vi "Get UI Refs.vi"(8 "error in (no error)":errorcluster, 11 "VI Refnum":refnum<vi>) -> (0 "error out":errorcluster, 3 "UI References":T1)   [LabVIEW 2018, in "Numeric Data Type.lvclass"]
uses:
  Numeric Data Type.lvclass
  UI References.ctl
  Representation Ring.ctl
  <vilib>/fxp/FXPxcontrol/FXP.xctl
  Response to Values Outside of Limits Enum.ctl
  Precision Type.ctl
  Padding.ctl
  Time Format.ctl
  Clock Type.ctl
  Date Format.ctl
  Date Order.ctl
  Year Format.ctl
  Format Code Type List Enum.ctl
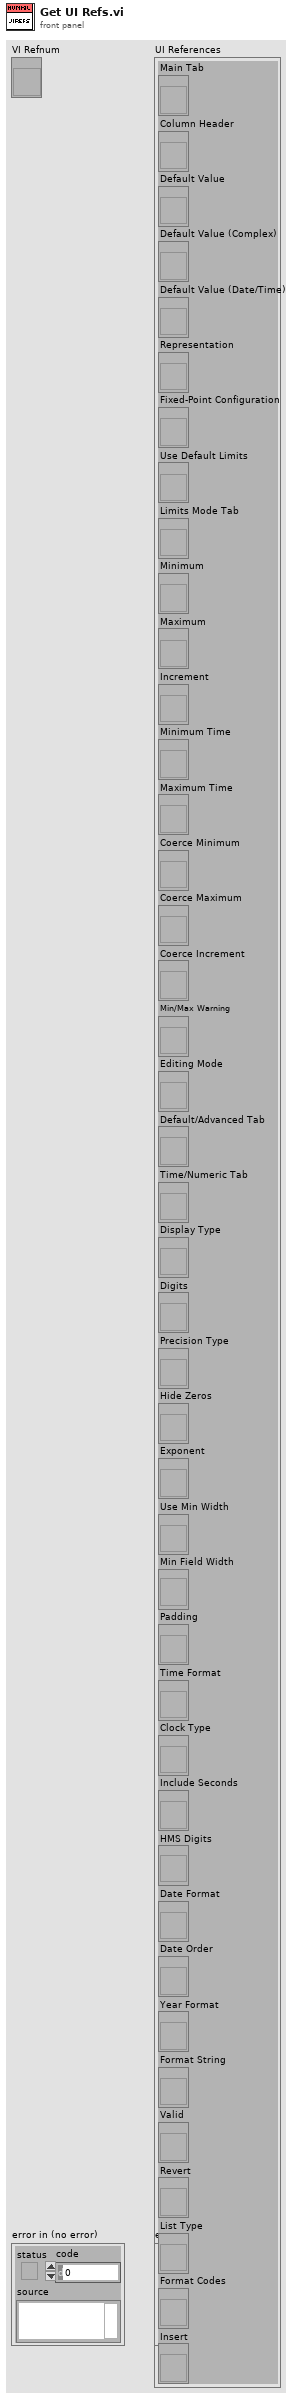
[diagram p1: front panel]
types:
  T1 = typedef "Numeric Data Type.lvclass/UI References.ctl" = cluster{"Main Tab":refnum<vi>, "Column Header":refnum<vi>, "Default Value":refnum<vi>, "Default Value (Complex)":refnum<vi>, "Default Value (Date/Time)":refnum<vi>, "Representation":refnum<vi>, "Fixed-Point Configuration":refnum<vi>, "Use Default Limits":refnum<vi>, "Limits Mode Tab":refnum<vi>, "Minimum":refnum<vi>, "Maximum":refnum<vi>, "Increment":refnum<vi>, "Minimum Time":refnum<vi>, "Maximum Time":refnum<vi>, "Coerce Minimum":refnum<vi>, "Coerce Maximum":refnum<vi>, "Coerce Increment":refnum<vi>, "Min/Max Warning":refnum<vi>, "Editing Mode":refnum<vi>, "Default/Advanced Tab":refnum<vi>, "Time/Numeric Tab":refnum<vi>, "Display Type":refnum<vi>, "Digits":refnum<vi>, "Precision Type":refnum<vi>, "Hide Zeros":refnum<vi>, "Exponent":refnum<vi>, "Use Min Width":refnum<vi>, "Min Field Width":refnum<vi>, "Padding":refnum<vi>, "Time Format":refnum<vi>, "Clock Type":refnum<vi>, "Include Seconds":refnum<vi>, "HMS Digits":refnum<vi>, "Date Format":refnum<vi>, "Date Order":refnum<vi>, "Year Format":refnum<vi>, "Format String":refnum<vi>, "Valid":refnum<vi>, "Revert":refnum<vi>, "List Type":refnum<vi>, "Format Codes":refnum<vi>, "Insert":refnum<vi>}
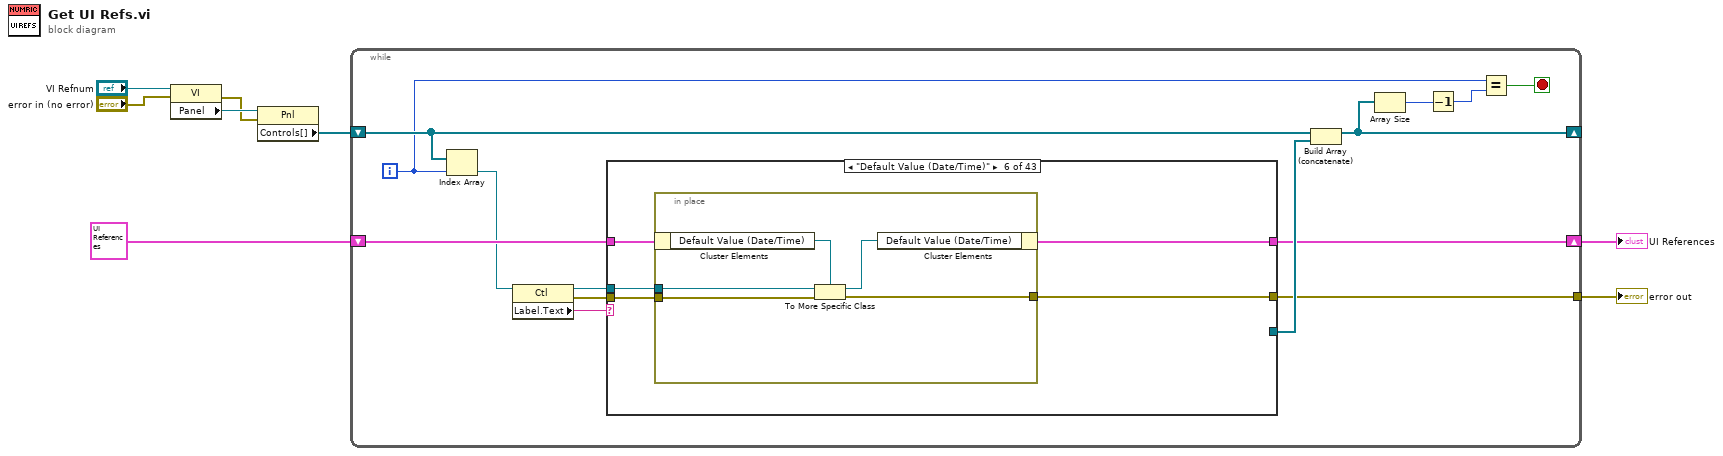
[diagram p0: block diagram]
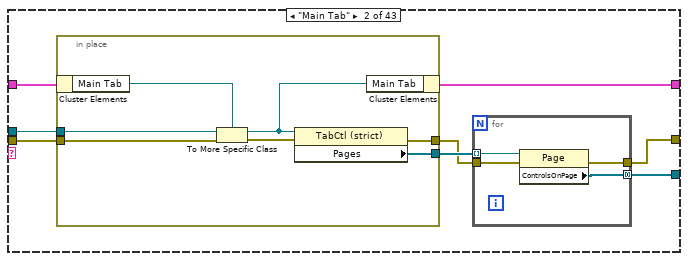
[diagram p3: hidden frame]
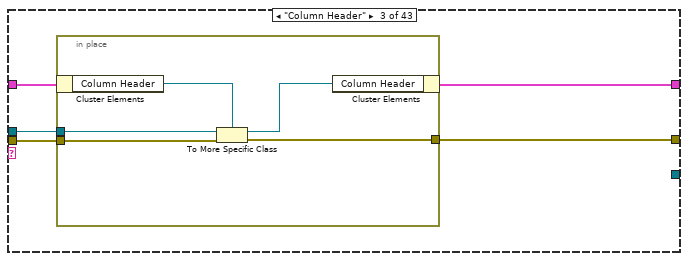
[diagram p4: hidden frame]
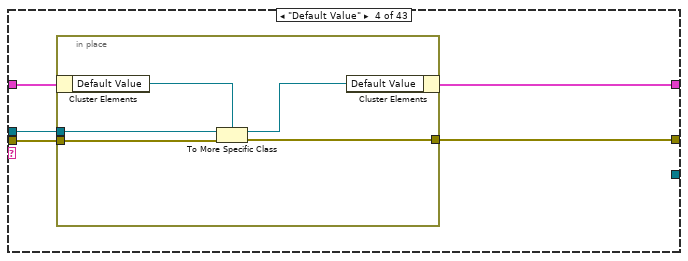
[diagram p5: hidden frame]
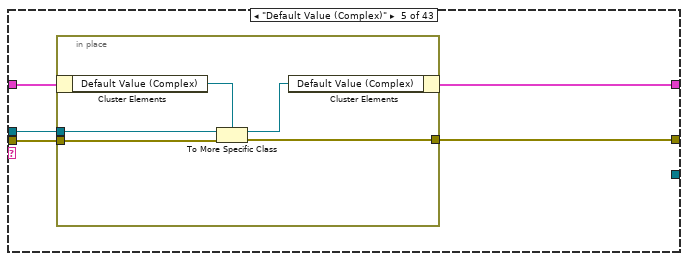
[diagram p6: hidden frame]
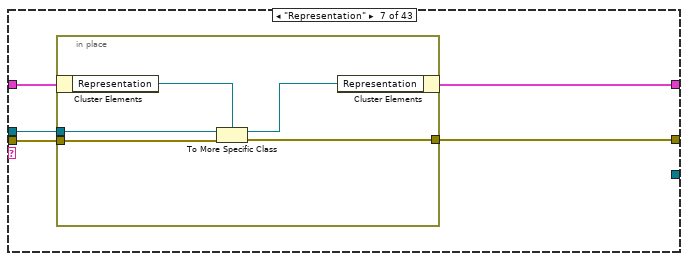
[diagram p7: hidden frame]
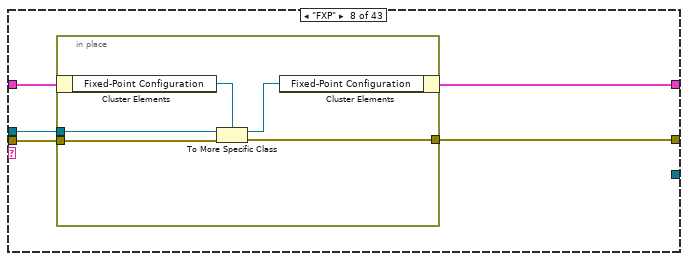
[diagram p8: hidden frame]
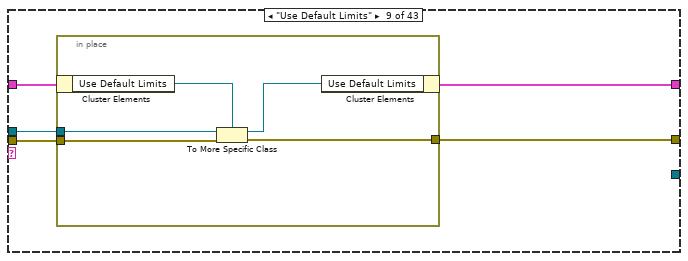
[diagram p9: hidden frame]
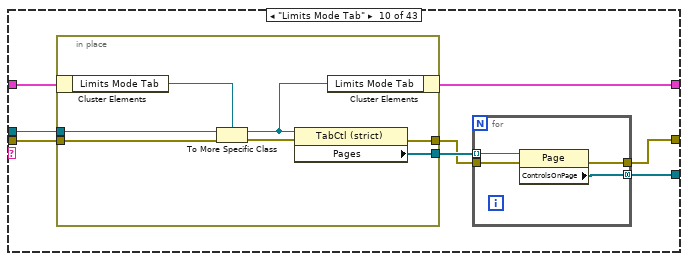
[diagram p10: hidden frame]
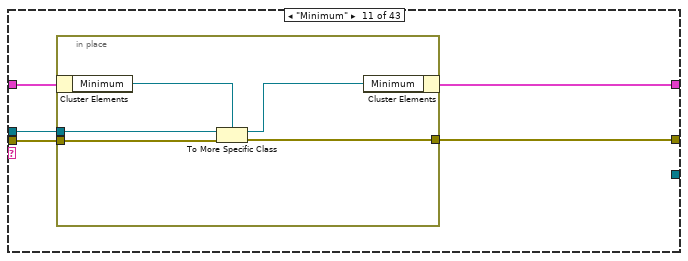
[diagram p11: hidden frame]
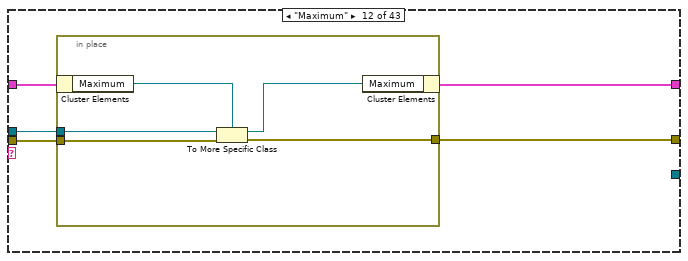
[diagram p12: hidden frame]
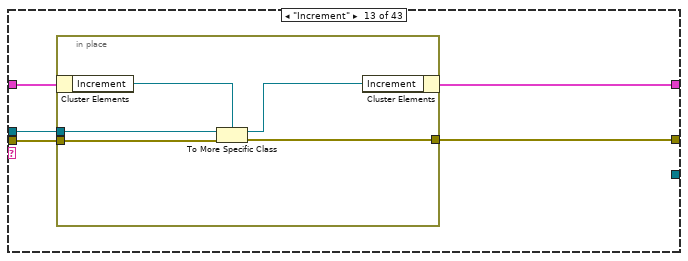
[diagram p13: hidden frame]
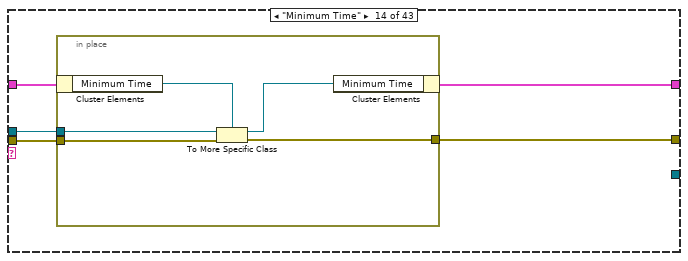
[diagram p14: hidden frame]
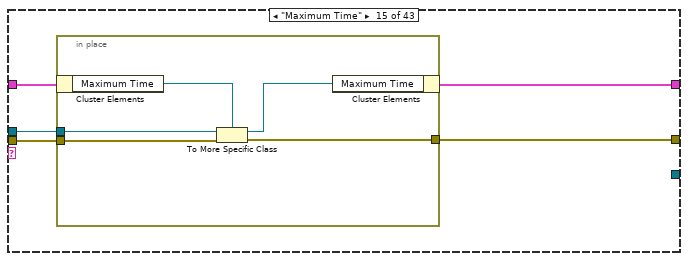
[diagram p15: hidden frame]
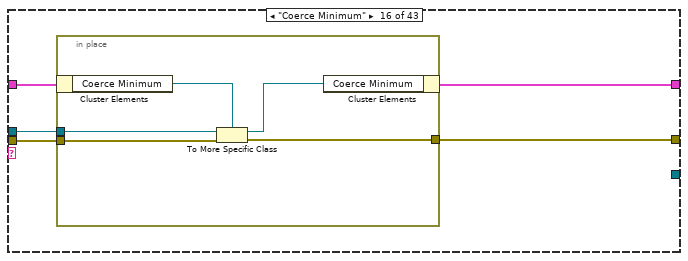
[diagram p16: hidden frame]
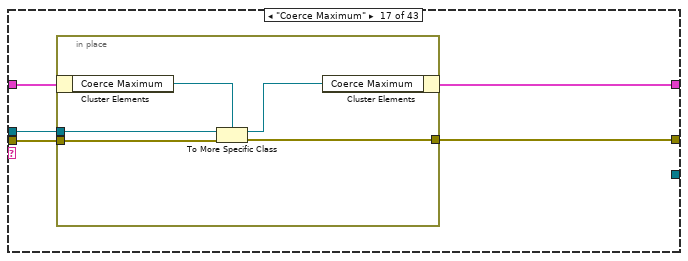
[diagram p17: hidden frame]
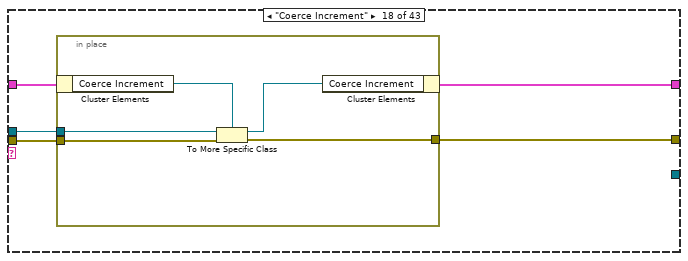
[diagram p18: hidden frame]
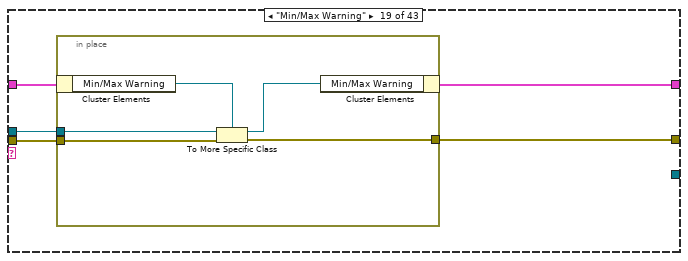
[diagram p19: hidden frame]
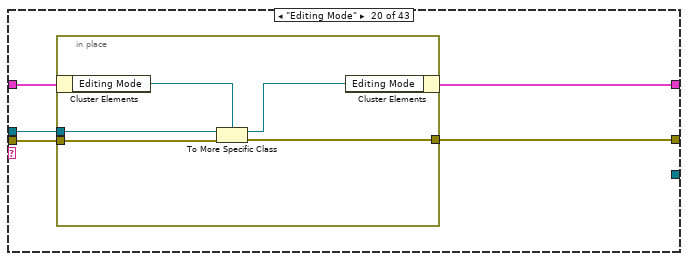
[diagram p20: hidden frame]
diagram:
  n1 = property class="VI"(reference="VI Refnum", error in="error in (no error)") -> (error out=w1:errorcluster, "Panel"=w4:refnum<vi>)  [unwired: 1 out]
  n2 = property class="Pnl"(reference=w4, error in=w1) -> ("Controls[]"=w3:refnum<vi>[])  [unwired: 2 out]
  n3 = while {
    shift-right: [w10] -> w6
    shift-left: T1 {"Main Tab"=refnum, "Column Header"=refnum, "Default Value"=refnum, "Default Value (Complex)"=refnum, "Default Value (Date/Time)"=refnum, "Representation"=refnum, "Fixed-Point Configuration"=refnum, "Use Default Limits"=refnum, "Limits Mode Tab"=refnum, "Minimum"=refnum, "Maximum"=refnum, "Increment"=refnum, "Minimum Time"=refnum, "Maximum Time"=refnum, "Coerce Minimum"=refnum, "Coerce Maximum"=refnum, "Coerce Increment"=refnum, "Min/Max Warning"=refnum, "Editing Mode"=refnum, "Default/Advanced Tab"=refnum, "Time/Numeric Tab"=refnum, "Display Type"=refnum, "Digits"=refnum, "Precision Type"=refnum, "Hide Zeros"=refnum, "Exponent"=refnum, "Use Min Width"=refnum, "Min Field Width"=refnum, "Padding"=refnum, "Time Format"=refnum, "Clock Type"=refnum, "Include Seconds"=refnum, "HMS Digits"=refnum, "Date Format"=refnum, "Date Order"=refnum, "Year Format"=refnum, "Format String"=refnum, "Valid"=refnum, "Revert"=refnum, "List Type"=refnum, "Format Codes"=refnum, "Insert"=refnum} ("UI References") -> [w22]
    shift-right: [w15] -> _
    shift-left: w3 -> [w17]
    tunnel: [w9] -> w8
    i -> [w13]
    stop <- w11 stop-if-true
    n4 = Index Array(array=w17, index=w13) -> (element=w21:refnum<vi>)
    n5 = property class="Ctl"(reference=w21) -> (reference out=w19:refnum<vi>, error out=w18:errorcluster, "Label.Text"=w20:string)  [unwired: 1 in]
    n6 = case shown="\"Default Value (Date/Time)\"" w20 {
      tunnel: w22 -> [w24 w31 w47 w57 w67 w77 w87 w97 w107 w120 w136 w146 w156 w166 w176 w186 w196 w206 w216 w226 w239 w258 w274 w284 w294 w304 w314 w324 w334 w344 w354 w364 w374 w384 w394 w404 w414 w424 w434 w444 w454 w464 w474]
      tunnel: w19 -> [_ w32 w48 w58 w68 w78 w88 w98 w108 w121 w137 w147 w157 w167 w177 w187 w197 w207 w217 w227 w240 w259 w275 w285 w295 w305 w315 w325 w335 w345 w355 w365 w375 w385 w395 w405 w415 w425 w435 w445 w455 w465 w475]
      tunnel: w18 -> [w23 w30 w46 w56 w66 w76 w86 w96 w106 w119 w135 w145 w155 w165 w175 w185 w195 w205 w215 w225 w238 w257 w273 w283 w293 w303 w313 w323 w333 w343 w353 w363 w373 w383 w393 w403 w413 w423 w433 w443 w453 w463 w473]
      tunnel: [_ w28 _ _ _ _ _ _ _ w117 _ _ _ _ _ _ _ _ _ _ w236 w255 _ _ _ _ _ _ _ _ _ _ _ _ _ _ _ _ _ _ _ _ _] -> w16
      tunnel: [w24 w27 w45 w55 w65 w75 w85 w95 w105 w116 w134 w144 w154 w164 w174 w184 w194 w204 w214 w224 w235 w254 w272 w282 w292 w302 w312 w322 w332 w342 w352 w362 w372 w382 w392 w402 w412 w422 w432 w442 w452 w462 w472] -> w10
      tunnel: [w23 w25 w44 w54 w64 w74 w84 w94 w104 w114 w133 w143 w153 w163 w173 w183 w193 w203 w213 w223 w233 w252 w271 w281 w291 w301 w311 w321 w331 w341 w351 w361 w371 w381 w391 w401 w411 w421 w431 w441 w451 w461 w471] -> w9
      frame Default {
      }
      frame "Main Tab" {
        n7 = in-place {
          in-place-border: w32 -> [w39]
          in-place-border: w30 -> [w37]
          in-place-border: [w34] -> w29
          in-place-border: [w33] -> w26
          n8 = in-place-cluster #1(w31) -> ("Main Tab"=w38:refnum<vi>)
          n9 = To More Specific Class(target class=w38, reference=w39, error in=w37) -> (specific class reference=w36:refnum<vi>, error out=w35:errorcluster)
          n10 = property class="TabCtl (strict)"(reference=w36, error in=w35) -> (error out=w33:errorcluster, "Pages"=w34:refnum<vi>[])  [unwired: 1 out]
          n11 = in-place-cluster #1("Main Tab"=w36) -> (w27:T1)
        }
        n12 = for {
          tunnel: w29 -> [w43] mode=indexing
          tunnel: [w42] -> w28 mode=concatenating
          tunnel: w26 -> [w41]
          tunnel: [w40] -> w25
          n13 = property class="Page"(reference=w43, error in=w41) -> (error out=w40:errorcluster, "ControlsOnPage"=w42:refnum<vi>[])  [unwired: 1 out]
        }
      }
      frame "Column Header" {
        n14 = in-place {
          in-place-border: w48 -> [w53]
          in-place-border: w46 -> [w51]
          in-place-border: [w49] -> w44
          n15 = in-place-cluster #2(w47) -> ("Column Header"=w52:refnum<vi>)
          n16 = To More Specific Class(target class=w52, reference=w53, error in=w51) -> (specific class reference=w50:refnum<vi>, error out=w49:errorcluster)
          n17 = in-place-cluster #2("Column Header"=w50) -> (w45:T1)
        }
      }
      frame "Default Value" {
        n18 = in-place {
          in-place-border: w58 -> [w63]
          in-place-border: w56 -> [w61]
          in-place-border: [w59] -> w54
          n19 = in-place-cluster #3(w57) -> ("Default Value"=w62:refnum<vi>)
          n20 = To More Specific Class(target class=w62, reference=w63, error in=w61) -> (specific class reference=w60:refnum<vi>, error out=w59:errorcluster)
          n21 = in-place-cluster #3("Default Value"=w60) -> (w55:T1)
        }
      }
      frame "Default Value (Complex)" {
        n22 = in-place {
          in-place-border: w68 -> [w73]
          in-place-border: w66 -> [w71]
          in-place-border: [w69] -> w64
          n23 = in-place-cluster #4(w67) -> ("Default Value (Complex)"=w72:refnum<vi>)
          n24 = To More Specific Class(target class=w72, reference=w73, error in=w71) -> (specific class reference=w70:refnum<vi>, error out=w69:errorcluster)
          n25 = in-place-cluster #4("Default Value (Complex)"=w70) -> (w65:T1)
        }
      }
      frame "Default Value (Date/Time)" {
        n26 = in-place {
          in-place-border: w78 -> [w83]
          in-place-border: w76 -> [w81]
          in-place-border: [w79] -> w74
          n27 = in-place-cluster #5(w77) -> ("Default Value (Date/Time)"=w82:refnum<vi>)
          n28 = To More Specific Class(target class=w82, reference=w83, error in=w81) -> (specific class reference=w80:refnum<vi>, error out=w79:errorcluster)
          n29 = in-place-cluster #5("Default Value (Date/Time)"=w80) -> (w75:T1)
        }
      }
      frame "Representation" {
        n30 = in-place {
          in-place-border: w88 -> [w93]
          in-place-border: w86 -> [w91]
          in-place-border: [w89] -> w84
          n31 = in-place-cluster #6(w87) -> ("Representation"=w92:refnum<vi>)
          n32 = To More Specific Class(target class=w92, reference=w93, error in=w91) -> (specific class reference=w90:refnum<vi>, error out=w89:errorcluster)
          n33 = in-place-cluster #6("Representation"=w90) -> (w85:T1)
        }
      }
      frame "FXP" {
        n34 = in-place {
          in-place-border: w98 -> [w103]
          in-place-border: w96 -> [w101]
          in-place-border: [w99] -> w94
          n35 = in-place-cluster #7(w97) -> ("Fixed-Point Configuration"=w102:refnum<vi>)
          n36 = To More Specific Class(target class=w102, reference=w103, error in=w101) -> (specific class reference=w100:refnum<vi>, error out=w99:errorcluster)
          n37 = in-place-cluster #7("Fixed-Point Configuration"=w100) -> (w95:T1)
        }
      }
      frame "Use Default Limits" {
        n38 = in-place {
          in-place-border: w108 -> [w113]
          in-place-border: w106 -> [w111]
          in-place-border: [w109] -> w104
          n39 = in-place-cluster #8(w107) -> ("Use Default Limits"=w112:refnum<vi>)
          n40 = To More Specific Class(target class=w112, reference=w113, error in=w111) -> (specific class reference=w110:refnum<vi>, error out=w109:errorcluster)
          n41 = in-place-cluster #8("Use Default Limits"=w110) -> (w105:T1)
        }
      }
      frame "Limits Mode Tab" {
        n42 = in-place {
          in-place-border: w121 -> [w128]
          in-place-border: w119 -> [w126]
          in-place-border: [w123] -> w118
          in-place-border: [w122] -> w115
          n43 = in-place-cluster #9(w120) -> ("Limits Mode Tab"=w127:refnum<vi>)
          n44 = To More Specific Class(target class=w127, reference=w128, error in=w126) -> (specific class reference=w125:refnum<vi>, error out=w124:errorcluster)
          n45 = property class="TabCtl (strict)"(reference=w125, error in=w124) -> (error out=w122:errorcluster, "Pages"=w123:refnum<vi>[])  [unwired: 1 out]
          n46 = in-place-cluster #9("Limits Mode Tab"=w125) -> (w116:T1)
        }
        n47 = for {
          tunnel: w118 -> [w132] mode=indexing
          tunnel: [w131] -> w117 mode=concatenating
          tunnel: w115 -> [w130]
          tunnel: [w129] -> w114
          n48 = property class="Page"(reference=w132, error in=w130) -> (error out=w129:errorcluster, "ControlsOnPage"=w131:refnum<vi>[])  [unwired: 1 out]
        }
      }
      frame "Minimum" {
        n49 = in-place {
          in-place-border: w137 -> [w142]
          in-place-border: w135 -> [w140]
          in-place-border: [w138] -> w133
          n50 = in-place-cluster #10(w136) -> ("Minimum"=w141:refnum<vi>)
          n51 = To More Specific Class(target class=w141, reference=w142, error in=w140) -> (specific class reference=w139:refnum<vi>, error out=w138:errorcluster)
          n52 = in-place-cluster #10("Minimum"=w139) -> (w134:T1)
        }
      }
      frame "Maximum" {
        n53 = in-place {
          in-place-border: w147 -> [w152]
          in-place-border: w145 -> [w150]
          in-place-border: [w148] -> w143
          n54 = in-place-cluster #11(w146) -> ("Maximum"=w151:refnum<vi>)
          n55 = To More Specific Class(target class=w151, reference=w152, error in=w150) -> (specific class reference=w149:refnum<vi>, error out=w148:errorcluster)
          n56 = in-place-cluster #11("Maximum"=w149) -> (w144:T1)
        }
      }
      frame "Increment" {
        n57 = in-place {
          in-place-border: w157 -> [w162]
          in-place-border: w155 -> [w160]
          in-place-border: [w158] -> w153
          n58 = in-place-cluster #12(w156) -> ("Increment"=w161:refnum<vi>)
          n59 = To More Specific Class(target class=w161, reference=w162, error in=w160) -> (specific class reference=w159:refnum<vi>, error out=w158:errorcluster)
          n60 = in-place-cluster #12("Increment"=w159) -> (w154:T1)
        }
      }
      frame "Minimum Time" {
        n61 = in-place {
          in-place-border: w167 -> [w172]
          in-place-border: w165 -> [w170]
          in-place-border: [w168] -> w163
          n62 = in-place-cluster #13(w166) -> ("Minimum Time"=w171:refnum<vi>)
          n63 = To More Specific Class(target class=w171, reference=w172, error in=w170) -> (specific class reference=w169:refnum<vi>, error out=w168:errorcluster)
          n64 = in-place-cluster #13("Minimum Time"=w169) -> (w164:T1)
        }
      }
      frame "Maximum Time" {
        n65 = in-place {
          in-place-border: w177 -> [w182]
          in-place-border: w175 -> [w180]
          in-place-border: [w178] -> w173
          n66 = in-place-cluster #14(w176) -> ("Maximum Time"=w181:refnum<vi>)
          n67 = To More Specific Class(target class=w181, reference=w182, error in=w180) -> (specific class reference=w179:refnum<vi>, error out=w178:errorcluster)
          n68 = in-place-cluster #14("Maximum Time"=w179) -> (w174:T1)
        }
      }
      frame "Coerce Minimum" {
        n69 = in-place {
          in-place-border: w187 -> [w192]
          in-place-border: w185 -> [w190]
          in-place-border: [w188] -> w183
          n70 = in-place-cluster #15(w186) -> ("Coerce Minimum"=w191:refnum<vi>)
          n71 = To More Specific Class(target class=w191, reference=w192, error in=w190) -> (specific class reference=w189:refnum<vi>, error out=w188:errorcluster)
          n72 = in-place-cluster #15("Coerce Minimum"=w189) -> (w184:T1)
        }
      }
      frame "Coerce Maximum" {
        n73 = in-place {
          in-place-border: w197 -> [w202]
          in-place-border: w195 -> [w200]
          in-place-border: [w198] -> w193
          n74 = in-place-cluster #16(w196) -> ("Coerce Maximum"=w201:refnum<vi>)
          n75 = To More Specific Class(target class=w201, reference=w202, error in=w200) -> (specific class reference=w199:refnum<vi>, error out=w198:errorcluster)
          n76 = in-place-cluster #16("Coerce Maximum"=w199) -> (w194:T1)
        }
      }
      frame "Coerce Increment" {
        n77 = in-place {
          in-place-border: w207 -> [w212]
          in-place-border: w205 -> [w210]
          in-place-border: [w208] -> w203
          n78 = in-place-cluster #17(w206) -> ("Coerce Increment"=w211:refnum<vi>)
          n79 = To More Specific Class(target class=w211, reference=w212, error in=w210) -> (specific class reference=w209:refnum<vi>, error out=w208:errorcluster)
          n80 = in-place-cluster #17("Coerce Increment"=w209) -> (w204:T1)
        }
      }
      frame "Min/Max Warning" {
        n81 = in-place {
          in-place-border: w217 -> [w222]
          in-place-border: w215 -> [w220]
          in-place-border: [w218] -> w213
          n82 = in-place-cluster #18(w216) -> ("Min/Max Warning"=w221:refnum<vi>)
          n83 = To More Specific Class(target class=w221, reference=w222, error in=w220) -> (specific class reference=w219:refnum<vi>, error out=w218:errorcluster)
          n84 = in-place-cluster #18("Min/Max Warning"=w219) -> (w214:T1)
        }
      }
      frame "Editing Mode" {
        n85 = in-place {
          in-place-border: w227 -> [w232]
          in-place-border: w225 -> [w230]
          in-place-border: [w228] -> w223
          n86 = in-place-cluster #19(w226) -> ("Editing Mode"=w231:refnum<vi>)
          n87 = To More Specific Class(target class=w231, reference=w232, error in=w230) -> (specific class reference=w229:refnum<vi>, error out=w228:errorcluster)
          n88 = in-place-cluster #19("Editing Mode"=w229) -> (w224:T1)
        }
      }
      frame "Default/Advanced Tab" {
        n89 = in-place {
          in-place-border: w240 -> [w247]
          in-place-border: w238 -> [w245]
          in-place-border: [w242] -> w237
          in-place-border: [w241] -> w234
          n90 = in-place-cluster #20(w239) -> ("Default/Advanced Tab"=w246:refnum<vi>)
          n91 = To More Specific Class(target class=w246, reference=w247, error in=w245) -> (specific class reference=w244:refnum<vi>, error out=w243:errorcluster)
          n92 = property class="TabCtl (strict)"(reference=w244, error in=w243) -> (error out=w241:errorcluster, "Pages"=w242:refnum<vi>[])  [unwired: 1 out]
          n93 = in-place-cluster #20("Default/Advanced Tab"=w244) -> (w235:T1)
        }
        n94 = for {
          tunnel: w237 -> [w251] mode=indexing
          tunnel: [w250] -> w236 mode=concatenating
          tunnel: w234 -> [w249]
          tunnel: [w248] -> w233
          n95 = property class="Page"(reference=w251, error in=w249) -> (error out=w248:errorcluster, "ControlsOnPage"=w250:refnum<vi>[])  [unwired: 1 out]
        }
      }
      frame "Time/Numeric Tab" {
        n96 = in-place {
          in-place-border: w259 -> [w266]
          in-place-border: w257 -> [w264]
          in-place-border: [w261] -> w256
          in-place-border: [w260] -> w253
          n97 = in-place-cluster #21(w258) -> ("Time/Numeric Tab"=w265:refnum<vi>)
          n98 = To More Specific Class(target class=w265, reference=w266, error in=w264) -> (specific class reference=w263:refnum<vi>, error out=w262:errorcluster)
          n99 = property class="TabCtl (strict)"(reference=w263, error in=w262) -> (error out=w260:errorcluster, "Pages"=w261:refnum<vi>[])  [unwired: 1 out]
          n100 = in-place-cluster #21("Time/Numeric Tab"=w263) -> (w254:T1)
        }
        n101 = for {
          tunnel: w256 -> [w270] mode=indexing
          tunnel: [w269] -> w255 mode=concatenating
          tunnel: w253 -> [w268]
          tunnel: [w267] -> w252
          n102 = property class="Page"(reference=w270, error in=w268) -> (error out=w267:errorcluster, "ControlsOnPage"=w269:refnum<vi>[])  [unwired: 1 out]
        }
      }
      frame "Type" {
        n103 = in-place {
          in-place-border: w275 -> [w280]
          in-place-border: w273 -> [w278]
          in-place-border: [w276] -> w271
          n104 = in-place-cluster #22(w274) -> ("Display Type"=w279:refnum<vi>)
          n105 = To More Specific Class(target class=w279, reference=w280, error in=w278) -> (specific class reference=w277:refnum<vi>, error out=w276:errorcluster)
          n106 = in-place-cluster #22("Display Type"=w277) -> (w272:T1)
        }
      }
      frame "Digits" {
        n107 = in-place {
          in-place-border: w285 -> [w290]
          in-place-border: w283 -> [w288]
          in-place-border: [w286] -> w281
          n108 = in-place-cluster #23(w284) -> ("Digits"=w289:refnum<vi>)
          n109 = To More Specific Class(target class=w289, reference=w290, error in=w288) -> (specific class reference=w287:refnum<vi>, error out=w286:errorcluster)
          n110 = in-place-cluster #23("Digits"=w287) -> (w282:T1)
        }
      }
      frame "Precision Type" {
        n111 = in-place {
          in-place-border: w295 -> [w300]
          in-place-border: w293 -> [w298]
          in-place-border: [w296] -> w291
          n112 = in-place-cluster #24(w294) -> ("Precision Type"=w299:refnum<vi>)
          n113 = To More Specific Class(target class=w299, reference=w300, error in=w298) -> (specific class reference=w297:refnum<vi>, error out=w296:errorcluster)
          n114 = in-place-cluster #24("Precision Type"=w297) -> (w292:T1)
        }
      }
      frame "Hide Zeroes" {
        n115 = in-place {
          in-place-border: w305 -> [w310]
          in-place-border: w303 -> [w308]
          in-place-border: [w306] -> w301
          n116 = in-place-cluster #25(w304) -> ("Hide Zeros"=w309:refnum<vi>)
          n117 = To More Specific Class(target class=w309, reference=w310, error in=w308) -> (specific class reference=w307:refnum<vi>, error out=w306:errorcluster)
          n118 = in-place-cluster #25("Hide Zeros"=w307) -> (w302:T1)
        }
      }
      frame "Exponent" {
        n119 = in-place {
          in-place-border: w315 -> [w320]
          in-place-border: w313 -> [w318]
          in-place-border: [w316] -> w311
          n120 = in-place-cluster #26(w314) -> ("Exponent"=w319:refnum<vi>)
          n121 = To More Specific Class(target class=w319, reference=w320, error in=w318) -> (specific class reference=w317:refnum<vi>, error out=w316:errorcluster)
          n122 = in-place-cluster #26("Exponent"=w317) -> (w312:T1)
        }
      }
      frame "Use Min Width" {
        n123 = in-place {
          in-place-border: w325 -> [w330]
          in-place-border: w323 -> [w328]
          in-place-border: [w326] -> w321
          n124 = in-place-cluster #27(w324) -> ("Use Min Width"=w329:refnum<vi>)
          n125 = To More Specific Class(target class=w329, reference=w330, error in=w328) -> (specific class reference=w327:refnum<vi>, error out=w326:errorcluster)
          n126 = in-place-cluster #27("Use Min Width"=w327) -> (w322:T1)
        }
      }
      frame "Min Field Width" {
        n127 = in-place {
          in-place-border: w335 -> [w340]
          in-place-border: w333 -> [w338]
          in-place-border: [w336] -> w331
          n128 = in-place-cluster #28(w334) -> ("Min Field Width"=w339:refnum<vi>)
          n129 = To More Specific Class(target class=w339, reference=w340, error in=w338) -> (specific class reference=w337:refnum<vi>, error out=w336:errorcluster)
          n130 = in-place-cluster #28("Min Field Width"=w337) -> (w332:T1)
        }
      }
      frame "Padding" {
        n131 = in-place {
          in-place-border: w345 -> [w350]
          in-place-border: w343 -> [w348]
          in-place-border: [w346] -> w341
          n132 = in-place-cluster #29(w344) -> ("Padding"=w349:refnum<vi>)
          n133 = To More Specific Class(target class=w349, reference=w350, error in=w348) -> (specific class reference=w347:refnum<vi>, error out=w346:errorcluster)
          n134 = in-place-cluster #29("Padding"=w347) -> (w342:T1)
        }
      }
      frame "Time Format" {
        n135 = in-place {
          in-place-border: w355 -> [w360]
          in-place-border: w353 -> [w358]
          in-place-border: [w356] -> w351
          n136 = in-place-cluster #30(w354) -> ("Time Format"=w359:refnum<vi>)
          n137 = To More Specific Class(target class=w359, reference=w360, error in=w358) -> (specific class reference=w357:refnum<vi>, error out=w356:errorcluster)
          n138 = in-place-cluster #30("Time Format"=w357) -> (w352:T1)
        }
      }
      frame "Clock Type" {
        n139 = in-place {
          in-place-border: w365 -> [w370]
          in-place-border: w363 -> [w368]
          in-place-border: [w366] -> w361
          n140 = in-place-cluster #31(w364) -> ("Clock Type"=w369:refnum<vi>)
          n141 = To More Specific Class(target class=w369, reference=w370, error in=w368) -> (specific class reference=w367:refnum<vi>, error out=w366:errorcluster)
          n142 = in-place-cluster #31("Clock Type"=w367) -> (w362:T1)
        }
      }
      frame "Include Seconds" {
        n143 = in-place {
          in-place-border: w375 -> [w380]
          in-place-border: w373 -> [w378]
          in-place-border: [w376] -> w371
          n144 = in-place-cluster #32(w374) -> ("Include Seconds"=w379:refnum<vi>)
          n145 = To More Specific Class(target class=w379, reference=w380, error in=w378) -> (specific class reference=w377:refnum<vi>, error out=w376:errorcluster)
          n146 = in-place-cluster #32("Include Seconds"=w377) -> (w372:T1)
        }
      }
      frame "HMS Digits" {
        n147 = in-place {
          in-place-border: w385 -> [w390]
          in-place-border: w383 -> [w388]
          in-place-border: [w386] -> w381
          n148 = in-place-cluster #33(w384) -> ("HMS Digits"=w389:refnum<vi>)
          n149 = To More Specific Class(target class=w389, reference=w390, error in=w388) -> (specific class reference=w387:refnum<vi>, error out=w386:errorcluster)
          n150 = in-place-cluster #33("HMS Digits"=w387) -> (w382:T1)
        }
      }
      frame "Date Format" {
        n151 = in-place {
          in-place-border: w395 -> [w400]
          in-place-border: w393 -> [w398]
          in-place-border: [w396] -> w391
          n152 = in-place-cluster #34(w394) -> ("Date Format"=w399:refnum<vi>)
          n153 = To More Specific Class(target class=w399, reference=w400, error in=w398) -> (specific class reference=w397:refnum<vi>, error out=w396:errorcluster)
          n154 = in-place-cluster #34("Date Format"=w397) -> (w392:T1)
        }
      }
      frame "Date Order" {
        n155 = in-place {
          in-place-border: w405 -> [w410]
          in-place-border: w403 -> [w408]
          in-place-border: [w406] -> w401
          n156 = in-place-cluster #35(w404) -> ("Date Order"=w409:refnum<vi>)
          n157 = To More Specific Class(target class=w409, reference=w410, error in=w408) -> (specific class reference=w407:refnum<vi>, error out=w406:errorcluster)
          n158 = in-place-cluster #35("Date Order"=w407) -> (w402:T1)
        }
      }
      frame "Year Format" {
        n159 = in-place {
          in-place-border: w415 -> [w420]
          in-place-border: w413 -> [w418]
          in-place-border: [w416] -> w411
          n160 = in-place-cluster #36(w414) -> ("Year Format"=w419:refnum<vi>)
          n161 = To More Specific Class(target class=w419, reference=w420, error in=w418) -> (specific class reference=w417:refnum<vi>, error out=w416:errorcluster)
          n162 = in-place-cluster #36("Year Format"=w417) -> (w412:T1)
        }
      }
      frame "Format String" {
        n163 = in-place {
          in-place-border: w425 -> [w430]
          in-place-border: w423 -> [w428]
          in-place-border: [w426] -> w421
          n164 = in-place-cluster #37(w424) -> ("Format String"=w429:refnum<vi>)
          n165 = To More Specific Class(target class=w429, reference=w430, error in=w428) -> (specific class reference=w427:refnum<vi>, error out=w426:errorcluster)
          n166 = in-place-cluster #37("Format String"=w427) -> (w422:T1)
        }
      }
      frame "Valid" {
        n167 = in-place {
          in-place-border: w435 -> [w440]
          in-place-border: w433 -> [w438]
          in-place-border: [w436] -> w431
          n168 = in-place-cluster #38(w434) -> ("Valid"=w439:refnum<vi>)
          n169 = To More Specific Class(target class=w439, reference=w440, error in=w438) -> (specific class reference=w437:refnum<vi>, error out=w436:errorcluster)
          n170 = in-place-cluster #38("Valid"=w437) -> (w432:T1)
        }
      }
      frame "Revert" {
        n171 = in-place {
          in-place-border: w445 -> [w450]
          in-place-border: w443 -> [w448]
          in-place-border: [w446] -> w441
          n172 = in-place-cluster #39(w444) -> ("Revert"=w449:refnum<vi>)
          n173 = To More Specific Class(target class=w449, reference=w450, error in=w448) -> (specific class reference=w447:refnum<vi>, error out=w446:errorcluster)
          n174 = in-place-cluster #39("Revert"=w447) -> (w442:T1)
        }
      }
      frame "List Type" {
        n175 = in-place {
          in-place-border: w455 -> [w460]
          in-place-border: w453 -> [w458]
          in-place-border: [w456] -> w451
          n176 = in-place-cluster #40(w454) -> ("List Type"=w459:refnum<vi>)
          n177 = To More Specific Class(target class=w459, reference=w460, error in=w458) -> (specific class reference=w457:refnum<vi>, error out=w456:errorcluster)
          n178 = in-place-cluster #40("List Type"=w457) -> (w452:T1)
        }
      }
      frame "Format Codes" {
        n179 = in-place {
          in-place-border: w465 -> [w470]
          in-place-border: w463 -> [w468]
          in-place-border: [w466] -> w461
          n180 = in-place-cluster #41(w464) -> ("Format Codes"=w469:refnum<vi>)
          n181 = To More Specific Class(target class=w469, reference=w470, error in=w468) -> (specific class reference=w467:refnum<vi>, error out=w466:errorcluster)
          n182 = in-place-cluster #41("Format Codes"=w467) -> (w462:T1)
        }
      }
      frame "Insert" {
        n183 = in-place {
          in-place-border: w475 -> [w480]
          in-place-border: w473 -> [w478]
          in-place-border: [w476] -> w471
          n184 = in-place-cluster #42(w474) -> ("Insert"=w479:refnum<vi>)
          n185 = To More Specific Class(target class=w479, reference=w480, error in=w478) -> (specific class reference=w477:refnum<vi>, error out=w476:errorcluster)
          n186 = in-place-cluster #42("Insert"=w477) -> (w472:T1)
        }
      }
    }
    n187 = Build Array (concatenate)(w17, w16) -> (w15:refnum<vi>[])
    n188 = Array Size(array=w15) -> (size(s)=w14:i32)
    n189 = Decrement(x=w14) -> (x-1=w12:i32)
    n190 = Equal?(x=w13, y=w12) -> (x = y?=w11:bool)
  }
  "error out" <- w8
  "UI References" <- w6
